vi "_Static Data (Func Global).vi"(7 "Function (Read)":enum16{"Read", "Write"}(ring), 8 "error in (no error)":errorcluster, 10 "Numeric (0)":i32, 11 "Numeric in":refnum<class "Numeric Test Object.lvclass">) -> (0 "error out":errorcluster, 2 "Numeric out":i32, 3 "Numeric out":refnum<class "Numeric Test Object.lvclass">)   [LabVIEW 2009, in "Numeric Test Object.lvclass"]
doc: "This vi uses a functional global to implement static data."
uses:
  Numeric Test Object.lvclass
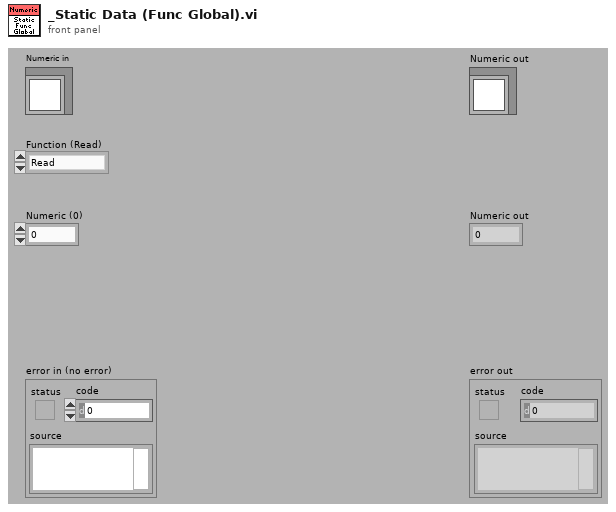
[diagram p1: front panel]
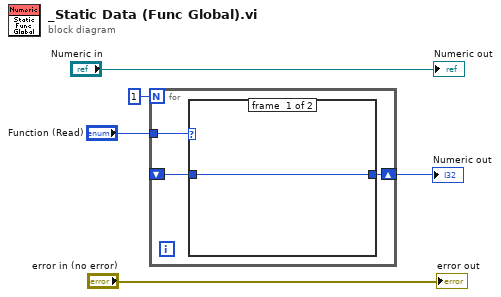
[diagram p0: block diagram]
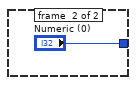
[diagram p2: hidden frame]
diagram:
  n1 = for {
    N: 1 -> [_]
    tunnel: "Function (Read)" -> [w8]
    shift-right: [w7] -> w1
    shift-left: _ -> [w6]
    n2 = case shown="\"Write\"" w8 {
      tunnel: [w9 "Numeric (0)"] -> w7
      tunnel: w6 -> [w9 _]
      frame #0 {
      }
      frame #1 {
      }
    }
  }
  "Numeric out" <- w1
  "error out" <- "error in (no error)"
  "Numeric out" <- "Numeric in"
